vi "Recieve Request for Result.vi"(6 "Request time":timestamp, 8 "error in (no error)":errorcluster, 9 "Requestor":string, 10 "Requestee":string, 11 "Compound Measurement in":refnum<class "Compound Measurement.lvclass">) -> (0 "error out":errorcluster, 3 "Compound Measurement out":refnum<class "Compound Measurement.lvclass">)   [LabVIEW 2015, in "Compound Measurement.lvclass"]
uses:
  Compound Measurement.lvclass
  Mag Lab Root/Mag Lab Root.lvclass/Mag Lab Root.ctl
  Compound Measurement.lvclass/Compound Measurement.ctl
  <vilib>/ActorFramework/Actor/Actor.lvclass/Actor.ctl
  <vilib>/ActorFramework/Message Enqueuer/Message Enqueuer.lvclass/Message Enqueuer.ctl
  Mag Lab Root Messages/Recieve Request for Result Msg/Recieve Request for Result Msg.lvclass/Recieve Request for Result Msg.ctl
  Write Awaiting Results.vi
  Write Finished.vi
  Mag Lab Root/Write Original requestor.vi
  <vilib>/ActorFramework/Message Enqueuer/Init from Existing Queue.vi
  <vilib>/ActorFramework/Message Enqueuer/Enqueue.vi
  <vilib>/ActorFramework/Message Priority Queue/Priority Enqueue.vi
  <vilib>/ActorFramework/Message Enqueuer/Message Enqueuer.lvclass
  Mag Lab Root Messages/Recieve Request for Result Msg/Recieve Request for Result Msg.lvclass
  <vilib>/ActorFramework/Actor/Actor.lvclass
  Mag Lab Root/Mag Lab Root.lvclass
  Mag Lab Error Handler/Mag Lab Error Handler.lvclass
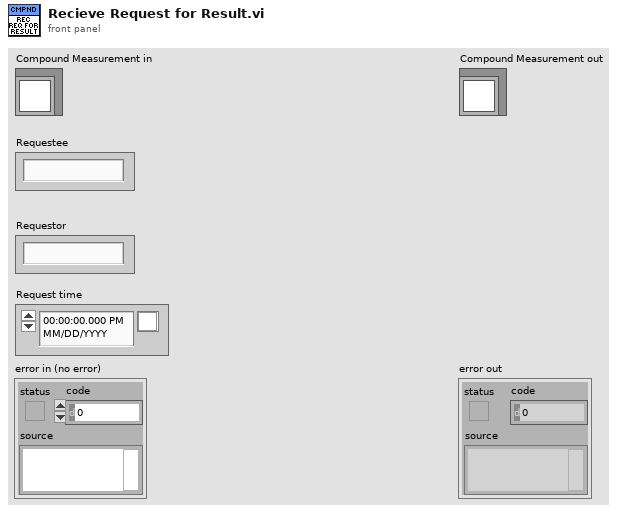
[diagram p1: front panel]
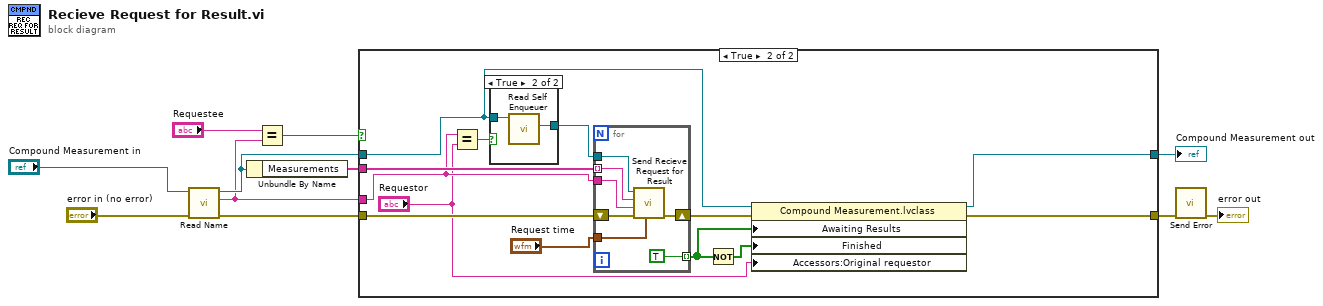
[diagram p0: block diagram]
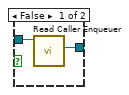
[diagram p3: hidden frame]
diagram:
  n1 = call "Read Name.vi"("error in (no error)"="error in (no error)", "Mag Lab Root in"="Compound Measurement in") -> ("error out"=w8:errorcluster, "Name"=w2:string, "Mag Lab Root out"=w5:refnum<class "Compound Measurement.lvclass">)  [unwired: 7 in]
  n2 = Unbundle By Name(w5) -> ("Measurements"=w11:string[])
  n3 = Equal?(x="Requestee", y=w2) -> (x = y?=w9:bool)
  n4 = case shown="True" w9 {
    tunnel: w11 -> [_ w26]
    tunnel: w5 -> [w13 w20]
    tunnel: [w12 w16] -> w7
    tunnel: [w13 w19] -> w10
    tunnel: w8 -> [w12 w24]
    tunnel: w2 -> [_ w23]
    frame False {
    }
    frame True {
      n5 = Equal?(x=w23, y="Requestor") -> (x = y?=w22:bool)
      n6 = case shown="True" w22 {
        tunnel: [w28 w29] -> w25
        tunnel: w20 -> [w27 w30]
        frame False {
          n7 = call <vilib>:"Read Caller Enqueuer.vi"("Actor"=w27) -> ("Caller Enqueuer"=w28:refnum<class "Message Enqueuer.lvclass">)  [unwired: 10 in]
        }
        frame True {
          n8 = call <vilib>:"Read Self Enqueuer.vi"("Actor"=w30) -> ("Self Enqueuer"=w29:refnum<class "Message Enqueuer.lvclass">)  [unwired: 10 in]
        }
      }
      n9 = for {
        tunnel: w26 -> [w36] mode=indexing
        tunnel: w23 -> [w37]
        shift-right: [w33] -> w17
        shift-left: w24 -> [w34]
        tunnel: w25 -> [w35]
        tunnel: [TRUE] -> w14 mode=indexing
        tunnel: "Request time" -> [w31]
        n10 = call "Send Recieve Request for Result.vi"("Request time"=w31, "error in (no error)"=w34, "Requestor"=w37, "Requestee"=w36, "Message Enqueuer"=w35) -> ("error out"=w33:errorcluster)  [unwired: 5 in, 1 out]
      }
      n11 = Not(x=w14) -> (.not. x?=w15:bool[])
      n12 = property class="Compound Measurement.lvclass"(reference=w20, error in=w17, "Awaiting Results"=w14, "Finished"=w15, "Accessors:Original requestor"="Requestor") -> (reference out=w19:refnum<class "Compound Measurement.lvclass">, error out=w16:errorcluster)
    }
  }
  "Compound Measurement out" <- w10
  n13 = call "Send Error.vi"("error in (no error)"=w7) -> ("error out"=→"error out":errorcluster)  [unwired: 9 in, 1 out]
